vi "OAT Polar PG Plot Polar Data.vi"(4 "polar attributes":T2 {"minimum" format="%.2f"; "maximum" format="%.2f"}, 5 "grid measurements":T1 {"end angle" format="%.2f"; "start angle" format="%.2f"; "scale factors"."b" format="%.2f"; "scale factors"."a" format="%.2f"}, 6 "polar data":cluster{"magnitude":dbl, "phase":dbl}[](array[cluster]) {"phase" format="%.2f"; "magnitude" format="%.2f"}, 7 "picture":picture) -> (3 "new picture":picture)   [LabVIEW 2017]
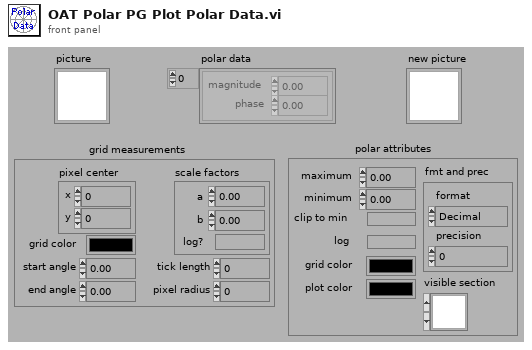
[diagram p1: front panel]
types:
  T1 = cluster{"pixel center":cluster{"x":i16, "y":i16}, "scale factors":cluster{"a":dbl, "b":dbl, "log?":bool}, "grid color":u32, "start angle":dbl, "end angle":dbl, "tick length":i16, "pixel radius":i32}
  T2 = cluster{"maximum":dbl, "minimum":dbl, "clip to min":bool, "log":bool, "grid color":u32, "plot color":u32, "fmt and prec":cluster{"format":enum8{"Decimal", "Scientific", "Engineering", "Binary", "Octal", "Hex"}, "precision":u8}, "visible section":u16}
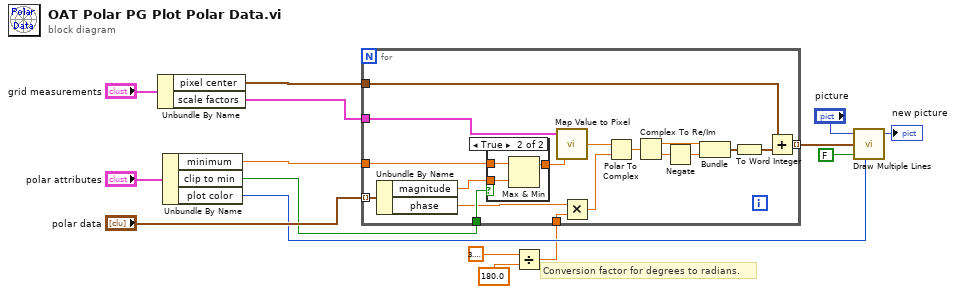
[diagram p0: block diagram]
diagram:
  # "Conversion factor for degrees to radians."
  n1 = Unbundle By Name("grid measurements") -> ("pixel center"=w7:cluster{"x":i16, "y":i16}, "scale factors"=w8:cluster{"a":dbl, "b":dbl, "log?":bool})
  n2 = Unbundle By Name("polar attributes") -> ("minimum"=w6:dbl, "clip to min"=w4:bool, "plot color"=w5:u32)
  n3 = Divide(x=3.141592653589793, y=180.0) -> (x/y=w2:dbl)
  n4 = for {
    tunnel: "polar data" -> [w33] mode=indexing
    tunnel: w7 -> [w32]
    tunnel: [w31] -> w11 mode=indexing
    tunnel: w8 -> [w24]
    tunnel: w6 -> [w20]
    tunnel: w4 -> [w19]
    tunnel: w2 -> [w16]
    n5 = Unbundle By Name(w33) -> ("magnitude"=w21:dbl, "phase"=w17:dbl)
    n6 = case shown="True" w19 {
      tunnel: w21 -> [w34 w37]
      tunnel: [w34 w36] -> w22
      tunnel: w20 -> [_ w35]
      frame False {
      }
      frame True {
        n7 = Max & Min(x=w35, y=w37) -> (max(x,y)=w36:dbl)  [unwired: 1 out]
      }
    }
    n8 = call <vilib>:"Map Value to Pixel.vi"("x"=w22, "scale factors"=w24) -> ("pixel"=w23:dbl)  [unwired: 1 in]
    n9 = Multiply(x=w17, y=w16) -> (x*y=w18:dbl)
    n10 = Polar To Complex(1:w18, 2:w23) -> (0:w30:cdb)
    n11 = Complex To Re/Im(x + iy=w30) -> (x=w28:dbl, y=w27:dbl)
    n12 = Negate(x=w27) -> (-x=w25:dbl)
    n13 = Bundle(w28, w25) -> (w29:cluster{dbl, dbl})  [unwired: 1 in]
    n14 = To Word Integer(number=w29) -> (16bit integer=w26:cluster{i16, i16})
    n15 = Add(x=w32, y=w26) -> (x+y=w31:cluster{i16, i16})
  }
  n16 = call <vilib>:"Draw Multiple Lines.vi"("picture"="picture", "line endpoints"=w11, "fill?(F)"=FALSE, "color(black)"=w5) -> ("new picture"=→"new picture":picture)  [unwired: 5 in]
